vi "Start Log.vi"(8 "Error In":errorcluster, 11 "Log Prefix":string) -> (0 "Error Out":errorcluster, 3 "refnum out":refnum<file>)   [LabVIEW 2015]
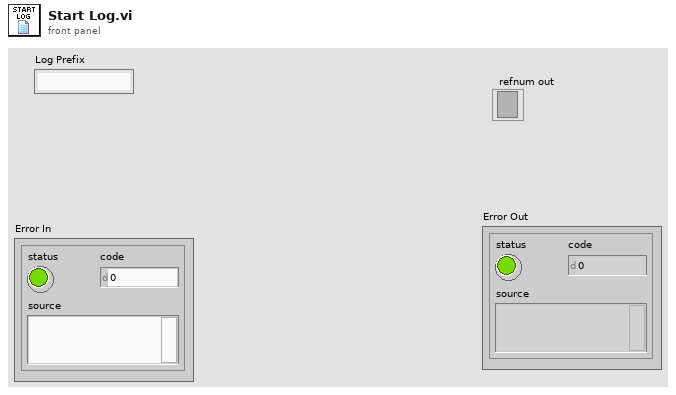
[diagram p1: front panel]
types:
  T1 = enum16{"open", "replace", "create", "open or create", "replace or create", "replace or create with confirmation"}
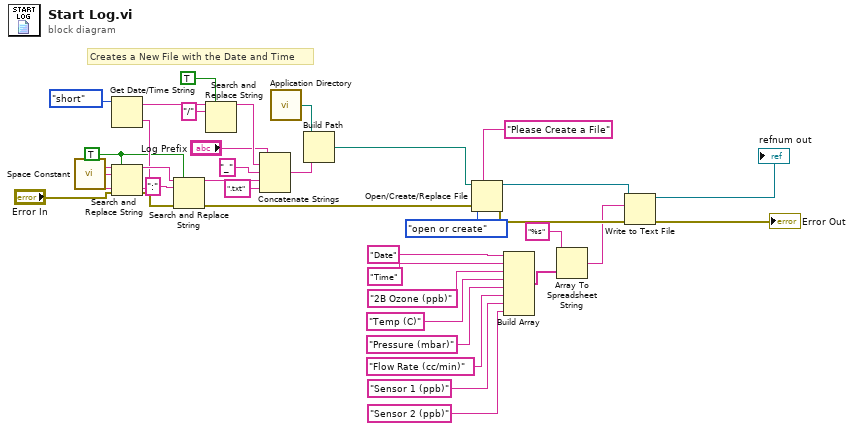
[diagram p0: block diagram]
diagram:
  w25 = TRUE
  # "Creates a New File with the Date and Time"
  n1 = call <vilib>:"Space Constant.vi"() -> ("String"=w28:string)
  n2 = Get Date/Time String(date format (0)=enum16{"short", "long", "abbreviated"}."short") -> (date string=w35:string, time string=w27:string)  [unwired: 2 in]
  n3 = Search and Replace String(replace all?=w25, input string=w27, search string=w28, error in="Error In") -> (result string=w33:string, error out=w11:errorcluster)  [unwired: 4 in, 2 out]
  n4 = Search and Replace String(replace all?=w25, input string=w33, search string=":", error in=w11) -> (result string=w26:string, error out=w10:errorcluster)  [unwired: 4 in, 2 out]
  n5 = Search and Replace String(replace all?=TRUE ("replace all? (F)"), input string=w35, search string="/") -> (result string=w29:string)  [unwired: 5 in, 3 out]
  n6 = Concatenate Strings("Log Prefix", w29, "_" ("string"), w26, ".txt" ("string")) -> (w37:string)
  n7 = call <vilib>:"Application Directory.vi"() -> ("Application Directory"=w23:path)
  n8 = Build Path(base path=w23, name or relative path=w37) -> (appended path=w14:path)
  n9 = Open/Create/Replace File(file path (use dialog)=w14, error in=w10, prompt="Please Create a File", operation (0:open)=T1."open or create") -> (refnum out=w21:refnum<file>, error out=w20:errorcluster)  [unwired: 2 in, 1 out]
  n10 = Build Array("Date", "Time", "2B Ozone (ppb)", "Temp (C)", "Pressure (mbar)", "Flow Rate (cc/min)", "Sensor 1 (ppb)", "Sensor 2 (ppb)") -> (w18:string[])
  n11 = Array To Spreadsheet String(array=w18, 3:"%s" ("format string")) -> (spreadsheet string=w17:string)  [unwired: 1 in]
  n12 = Write to Text File(file (use dialog)=w21, text=w17, error in=w20) -> (refnum out=→"refnum out":refnum<file>, error out=→"Error Out":errorcluster)  [unwired: 1 in, 1 out]
